vi "match_numbers.vi"() -> ()   [LabVIEW 2021]
panel:
  out "results":string[](array[string])
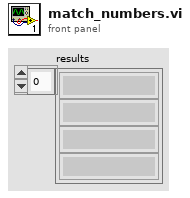
[diagram p1: front panel]
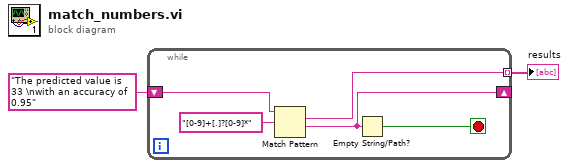
[diagram p0: block diagram]
diagram:
  n1 = while {
    shift-right: [w4] -> _
    shift-left: "The predicted value is 33 \nwith an accuracy of 0.95" -> [w7]
    tunnel: [w5] -> w1 mode=indexing
    stop <- w3 stop-if-true
    n2 = Match Pattern(string=w7, regular expression="[0-9]+[.]?[0-9]*") -> (match substring=w5:string, after substring=w4:string)  [unwired: 1 in, 2 out]
    n3 = Empty String/Path?(string/path=w4) -> (empty?=w3:bool)
  }
  "results" <- w1
